vi "Lab Panel V4.82.vi"() -> ()   [LabVIEW 2013] (continued)
                        n628 = Create Folder(path (use dialog)=w999) -> (error out=w998:errorcluster)  [unwired: 2 in, 2 out]
                        n629 = global write "Global 1.vi" "LAB03-1 FILE"(w985) -> ()
                        n630 = call <vilib>:"Clear Errors.vi"("error in (no error)"=w998) -> ()  [unwired: 6 in, 1 out]
                      }
                      frame #1 {
                        n631 = String To Path(string=w1010) -> (path=w1005:path)
                        n632 = TDMS Open(5:FALSE, 6:FALSE, 10:T19."create or replace" ("operation (0:open)"), 11:w1005) -> (0:w1004:errorcluster, 3:→"TDMS LAB03-1":refnum<k34>)  [unwired: 3 in]
                      }
                      frame #2 {
                        n633 = local read "SET LAB03-1"() -> (w1016:T5)
                        n634 = local read "TDMS LAB03-1"() -> (w1027:refnum<k34>)
                        n635 = Build Array("Testers Name", "Description", "Set Test Cycles", "T-Rise minutes", "T-Rise Deg C") -> (w1017:string[])
                        n636 = Unbundle(w1016) -> ("NAME"=w1015:string, "DESCRIPTION"=w1014:string, "CYCLES"=w1013:dbl, "T-RISE mins"=w1012:dbl, "T-RISE deg C"=w1011:dbl)
                        n637 = Number To Decimal String(number=w1013) -> (decimal integer string=w1026:string)  [unwired: 1 in]
                        n638 = Number To Decimal String(number=w1012) -> (decimal integer string=w1025:string)  [unwired: 1 in]
                        n639 = Number To Decimal String(number=w1011) -> (decimal integer string=w1024:string)  [unwired: 1 in]
                        n640 = Build Array(w1015, w1014, w1026, w1025, w1024) -> (w1023:string[])
                        n641 = TDMS Set Properties(5:w1023, 7:w1017, 11:w1027) -> ()  [unwired: 3 in, 4 out]
                      }
                      frame #3 {
                        w1029 = 0.0
                        n642 = local read "DISP LAB03-1"() -> (w1031:T4)
                        n643 = Bundle(cluster=w1031, "CYCLE"=w1029, "MINS"=w1029, "STATUS"="RUN") -> (w1030:T4)
                        n644 = local write "DISP LAB03-1"(w1030) -> ()
                      }
                      frame #4 {
                        n645 = local read "SIG LAB03-1"() -> (w1034:T2)
                        n646 = local read "TEMP START LAB03-1"() -> (w1036:cluster{"TL":dbl, "TN":dbl})
                        n647 = Unbundle(w1034) -> ("Tmp Live"=w1033:dbl, "Tmp Neut"=w1032:dbl)  [unwired: 3 out]
                        n648 = Bundle(cluster=w1036, "TL"=w1033, "TN"=w1032) -> (w1035:cluster{"TL":dbl, "TN":dbl})
                        n649 = local write "TEMP START LAB03-1"(w1035) -> ()
                      }
                    }
                  }
                }
              }
              event "RUN LAB03-2": Value Change {
                n650 = event-data() -> ("NewVal"=w1037:bool)  [unwired: 1 in, 5 out]
                n651 = local write "run lab03-2"(w1037) -> ()
                n652 = case shown="True" w1037 {
                  tunnel: w1043 -> [_ w1076]
                  tunnel: w1042 -> [_ w1075]
                  tunnel: w1040 -> [w1045 w1074]
                  tunnel: w1041 -> [_ w1073]
                  tunnel: w1039 -> [_ w1072]
                  tunnel: [w1044 w1071] -> w1038
                  frame False {
                    # "stop test"
                    n653 = stacked-sequence {
                      tunnel: w1045 -> [w1054 _]
                      tunnel: [w1046 _] -> w1044
                      frame #0 {
                        n654 = local read "DISP LAB03-2"() -> (w1053:T4)
                        n655 = Unbundle(w1053) -> ("CYCLE"=w1051:dbl, "MINS"=w1052:dbl)  [unwired: 1 out]
                        n656 = case shown="\"CYCLE TEST\"" w1054 {
                          tunnel: w1052 -> [_ _ w1061]
                          tunnel: w1051 -> [w1059 w1060 _]
                          tunnel: [w1059 w1060 w1061] -> w1050
                          frame "CHART TEST", Default {
                          }
                          frame "CYCLE TEST" {
                          }
                          frame "T-RISE TEST" {
                          }
                        }
                        n657 = local read "TDMS LAB03-2"() -> (w1058:refnum<k34>)
                        n658 = Build Array("STOPPED") -> (w1055:string[])
                        n659 = Build Array(w1050) -> (w1049:dbl[])
                        n660 = TDMS Write(0:w1058, 5:"TEST RESULT", 7:w1055, 9:w1049) -> (4:w1047:refnum<k34>, 15:w1048:errorcluster)  [unwired: 2 in, 2 out]
                        n661 = TDMS Close(8:w1048, 11:w1047) -> (0:w1046:errorcluster)  [unwired: 1 out]
                      }
                      frame #1 {
                        n662 = local read "DISP LAB03-2"() -> (w1065:T4)
                        n663 = stacked-sequence {
                          tunnel: "LAB03-2" -> [w1067 w1069]
                          frame #0 {
                            n664 = call "sub vi - defrag tdms v1.vi"("panel id"=w1067) -> ("error out"=w1066:errorcluster)  [unwired: 10 in]
                            n665 = local write "data file error"(w1066) -> ()
                          }
                          frame #1 {
                            n666 = call "Save data file to network drive v1.vi"("panel id"=w1069) -> ("network file save error"=w1068:errorcluster)  [unwired: 9 in, 1 out]
                            n667 = local write "RESULT LAB03-2"(FALSE) -> ()
                            n668 = local write "data file error"(w1068) -> ()
                          }
                        }
                        n669 = Bundle(cluster=w1065, "STATUS"="STOP") -> (w1063:T4)  [unwired: 2 in]
                        n670 = local write "DISP LAB03-2"(w1063) -> ()
                      }
                    }
                  }
                  frame True {
                    # "start new test and create test file"
                    n671 = stacked-sequence {
                      seq-local: [w1077 _ _ _ _] -> [_ w1102 _ _ _]
                      tunnel: w1076 -> [w1082 _ _ _ _]
                      tunnel: w1075 -> [w1079 _ _ _ _]
                      tunnel: w1074 -> [w1092 _ _ _ _]
                      tunnel: w1073 -> [w1085 _ _ _ _]
                      tunnel: w1072 -> [w1080 _ _ _ _]
                      tunnel: [_ w1096 _ _ _] -> w1071
                      frame #0 {
                        w1078 = "\\"
                        n672 = local read "SET LAB03-2"() -> (w1087:T5)
                        n673 = case shown="\"T-RISE TEST\"" w1092 {
                          tunnel: ["L03-2-CHART TEST-" "L03-2-CYCLE TEST-" "L03-2-T-RISE TEST-"] -> w1088
                          frame "CHART TEST", Default {
                          }
                          frame "CYCLE TEST" {
                          }
                          frame "T-RISE TEST" {
                          }
                        }
                        n674 = Unbundle(w1087) -> ("DESCRIPTION"=w1086:string)  [unwired: 4 out]
                        n675 = Concatenate Strings(w1082, "\\", w1080, w1078, w1079, w1078) -> (w1089:string)
                        n676 = String To Path(string=w1089) -> (path=w1091:path)
                        n677 = Concatenate Strings(w1089, w1088, w1086, "-", w1085, ".tdms") -> (w1077:string)
                        n678 = Create Folder(path (use dialog)=w1091) -> (error out=w1090:errorcluster)  [unwired: 2 in, 2 out]
                        n679 = global write "Global 1.vi" "LAB03-2 FILE"(w1077) -> ()
                        n680 = call <vilib>:"Clear Errors.vi"("error in (no error)"=w1090) -> ()  [unwired: 6 in, 1 out]
                      }
                      frame #1 {
                        n681 = String To Path(string=w1102) -> (path=w1097:path)
                        n682 = TDMS Open(5:FALSE, 6:FALSE, 10:T19."create or replace" ("operation (0:open)"), 11:w1097) -> (0:w1096:errorcluster, 3:→"TDMS LAB03-2":refnum<k34>)  [unwired: 3 in]
                      }
                      frame #2 {
                        n683 = local read "SET LAB03-2"() -> (w1108:T5)
                        n684 = local read "TDMS LAB03-2"() -> (w1119:refnum<k34>)
                        n685 = Build Array("Testers Name", "Description", "Set Test Cycles", "T-Rise minutes", "T-Rise Deg C") -> (w1109:string[])
                        n686 = Unbundle(w1108) -> ("NAME"=w1107:string, "DESCRIPTION"=w1106:string, "CYCLES"=w1105:dbl, "T-RISE mins"=w1104:dbl, "T-RISE deg C"=w1103:dbl)
                        n687 = Number To Decimal String(number=w1105) -> (decimal integer string=w1118:string)  [unwired: 1 in]
                        n688 = Number To Decimal String(number=w1104) -> (decimal integer string=w1117:string)  [unwired: 1 in]
                        n689 = Number To Decimal String(number=w1103) -> (decimal integer string=w1116:string)  [unwired: 1 in]
                        n690 = Build Array(w1107, w1106, w1118, w1117, w1116) -> (w1115:string[])
                        n691 = TDMS Set Properties(5:w1115, 7:w1109, 11:w1119) -> ()  [unwired: 3 in, 4 out]
                      }
                      frame #3 {
                        w1121 = 0.0
                        n692 = local read "DISP LAB03-2"() -> (w1123:T4)
                        n693 = Bundle(cluster=w1123, "CYCLE"=w1121, "MINS"=w1121, "STATUS"="RUN") -> (w1122:T4)
                        n694 = local write "DISP LAB03-2"(w1122) -> ()
                      }
                      frame #4 {
                        n695 = local read "SIG LAB03-2"() -> (w1126:T2)
                        n696 = local read "TEMP START LAB03-2"() -> (w1128:cluster{"TL":dbl, "TN":dbl})
                        n697 = Unbundle(w1126) -> ("Tmp Live"=w1125:dbl, "Tmp Neut"=w1124:dbl)  [unwired: 3 out]
                        n698 = Bundle(cluster=w1128, "TL"=w1125, "TN"=w1124) -> (w1127:cluster{"TL":dbl, "TN":dbl})
                        n699 = local write "TEMP START LAB03-2"(w1127) -> ()
                      }
                    }
                  }
                }
              }
              event "RUN LAB04-1": Value Change {
                n700 = event-data() -> ("NewVal"=w1129:bool)  [unwired: 1 in, 5 out]
                n701 = local write "run lab04-1"(w1129) -> ()
                n702 = case shown="True" w1129 {
                  tunnel: w1135 -> [_ w1168]
                  tunnel: w1134 -> [_ w1167]
                  tunnel: w1132 -> [w1137 w1166]
                  tunnel: w1133 -> [_ w1165]
                  tunnel: w1131 -> [_ w1164]
                  tunnel: [w1136 w1163] -> w1130
                  frame False {
                    # "stop test"
                    n703 = stacked-sequence {
                      tunnel: w1137 -> [w1146 _]
                      tunnel: [w1138 _] -> w1136
                      frame #0 {
                        n704 = local read "DISP LAB04-1"() -> (w1145:T4)
                        n705 = Unbundle(w1145) -> ("CYCLE"=w1143:dbl, "MINS"=w1144:dbl)  [unwired: 1 out]
                        n706 = case shown="\"CYCLE TEST\"" w1146 {
                          tunnel: w1144 -> [_ _ w1153]
                          tunnel: w1143 -> [w1151 w1152 _]
                          tunnel: [w1151 w1152 w1153] -> w1142
                          frame "CHART TEST", Default {
                          }
                          frame "CYCLE TEST" {
                          }
                          frame "T-RISE TEST" {
                          }
                        }
                        n707 = local read "TDMS LAB04-1"() -> (w1150:refnum<k34>)
                        n708 = Build Array("STOPPED") -> (w1147:string[])
                        n709 = Build Array(w1142) -> (w1141:dbl[])
                        n710 = TDMS Write(0:w1150, 5:"TEST RESULT", 7:w1147, 9:w1141) -> (4:w1139:refnum<k34>, 15:w1140:errorcluster)  [unwired: 2 in, 2 out]
                        n711 = TDMS Close(8:w1140, 11:w1139) -> (0:w1138:errorcluster)  [unwired: 1 out]
                      }
                      frame #1 {
                        n712 = local read "DISP LAB04-1"() -> (w1157:T4)
                        n713 = stacked-sequence {
                          tunnel: "LAB04-1" -> [w1159 w1161]
                          frame #0 {
                            n714 = call "sub vi - defrag tdms v1.vi"("panel id"=w1159) -> ("error out"=w1158:errorcluster)  [unwired: 10 in]
                            n715 = local write "data file error"(w1158) -> ()
                          }
                          frame #1 {
                            n716 = call "Save data file to network drive v1.vi"("panel id"=w1161) -> ("network file save error"=w1160:errorcluster)  [unwired: 9 in, 1 out]
                            n717 = local write "RESULT LAB04-1"(FALSE) -> ()
                            n718 = local write "data file error"(w1160) -> ()
                          }
                        }
                        n719 = Bundle(cluster=w1157, "STATUS"="STOP") -> (w1155:T4)  [unwired: 2 in]
                        n720 = local write "DISP LAB04-1"(w1155) -> ()
                      }
                    }
                  }
                  frame True {
                    # "start new test and create test file"
                    n721 = stacked-sequence {
                      seq-local: [w1169 _ _ _ _] -> [_ w1194 _ _ _]
                      tunnel: w1168 -> [w1174 _ _ _ _]
                      tunnel: w1167 -> [w1170 _ _ _ _]
                      tunnel: w1166 -> [w1184 _ _ _ _]
                      tunnel: w1165 -> [w1177 _ _ _ _]
                      tunnel: w1164 -> [w1172 _ _ _ _]
                      tunnel: [_ w1188 _ _ _] -> w1163
                      frame #0 {
                        w1171 = "\\"
                        n722 = local read "SET LAB04-1"() -> (w1179:T5)
                        n723 = case shown="\"CYCLE TEST\"" w1184 {
                          tunnel: ["L04-1-CHART TEST-" "L04-1-CYCLE TEST-" "L04-1-T-RISE TEST-"] -> w1180
                          frame "CHART TEST", Default {
                          }
                          frame "CYCLE TEST" {
                          }
                          frame "T-RISE TEST" {
                          }
                        }
                        n724 = Unbundle(w1179) -> ("DESCRIPTION"=w1178:string)  [unwired: 4 out]
                        n725 = Concatenate Strings(w1174, "\\", w1172, w1171, w1170, w1171) -> (w1181:string)
                        n726 = String To Path(string=w1181) -> (path=w1183:path)
                        n727 = Concatenate Strings(w1181, w1180, w1178, "-", w1177, ".tdms") -> (w1169:string)
                        n728 = Create Folder(path (use dialog)=w1183) -> (error out=w1182:errorcluster)  [unwired: 2 in, 2 out]
                        n729 = global write "Global 1.vi" "LAB04-1 FILE"(w1169) -> ()
                        n730 = call <vilib>:"Clear Errors.vi"("error in (no error)"=w1182) -> ()  [unwired: 6 in, 1 out]
                      }
                      frame #1 {
                        n731 = String To Path(string=w1194) -> (path=w1189:path)
                        n732 = TDMS Open(5:FALSE, 6:FALSE, 10:T19."create or replace" ("operation (0:open)"), 11:w1189) -> (0:w1188:errorcluster, 3:→"TDMS LAB04-1":refnum<k34>)  [unwired: 3 in]
                      }
                      frame #2 {
                        n733 = local read "SET LAB04-1"() -> (w1200:T5)
                        n734 = local read "TDMS LAB04-1"() -> (w1211:refnum<k34>)
                        n735 = Build Array("Testers Name", "Description", "Set Test Cycles", "T-Rise minutes", "T-Rise Deg C") -> (w1201:string[])
                        n736 = Unbundle(w1200) -> ("NAME"=w1199:string, "DESCRIPTION"=w1198:string, "CYCLES"=w1197:dbl, "T-RISE mins"=w1196:dbl, "T-RISE deg C"=w1195:dbl)
                        n737 = Number To Decimal String(number=w1197) -> (decimal integer string=w1210:string)  [unwired: 1 in]
                        n738 = Number To Decimal String(number=w1196) -> (decimal integer string=w1209:string)  [unwired: 1 in]
                        n739 = Number To Decimal String(number=w1195) -> (decimal integer string=w1208:string)  [unwired: 1 in]
                        n740 = Build Array(w1199, w1198, w1210, w1209, w1208) -> (w1207:string[])
                        n741 = TDMS Set Properties(5:w1207, 7:w1201, 11:w1211) -> ()  [unwired: 3 in, 4 out]
                      }
                      frame #3 {
                        w1213 = 0.0
                        n742 = local read "DISP LAB04-1"() -> (w1215:T4)
                        n743 = Bundle(cluster=w1215, "CYCLE"=w1213, "MINS"=w1213, "STATUS"="RUN") -> (w1214:T4)
                        n744 = local write "DISP LAB04-1"(w1214) -> ()
                      }
                      frame #4 {
                        n745 = local read "SIG LAB04-1"() -> (w1218:T2)
                        n746 = local read "TEMP START LAB04-1"() -> (w1220:cluster{"TL":dbl, "TN":dbl})
                        n747 = Unbundle(w1218) -> ("Tmp Live"=w1217:dbl, "Tmp Neut"=w1216:dbl)  [unwired: 3 out]
                        n748 = Bundle(cluster=w1220, "TL"=w1217, "TN"=w1216) -> (w1219:cluster{"TL":dbl, "TN":dbl})
                        n749 = local write "TEMP START LAB04-1"(w1219) -> ()
                      }
                    }
                  }
                }
              }
              event "RUN LAB04-2": Value Change {
                n750 = event-data() -> ("NewVal"=w1221:bool)  [unwired: 1 in, 5 out]
                n751 = local write "run lab04-2"(w1221) -> ()
                n752 = case shown="True" w1221 {
                  tunnel: w1227 -> [_ w1260]
                  tunnel: w1226 -> [_ w1259]
                  tunnel: w1224 -> [w1229 w1258]
                  tunnel: w1225 -> [_ w1257]
                  tunnel: w1223 -> [_ w1256]
                  tunnel: [w1228 w1255] -> w1222
                  frame False {
                    # "stop test"
                    n753 = stacked-sequence {
                      tunnel: w1229 -> [w1238 _]
                      tunnel: [w1230 _] -> w1228
                      frame #0 {
                        n754 = local read "DISP LAB04-2"() -> (w1237:T4)
                        n755 = Unbundle(w1237) -> ("CYCLE"=w1235:dbl, "MINS"=w1236:dbl)  [unwired: 1 out]
                        n756 = case shown="\"CYCLE TEST\"" w1238 {
                          tunnel: w1236 -> [_ _ w1245]
                          tunnel: w1235 -> [w1243 w1244 _]
                          tunnel: [w1243 w1244 w1245] -> w1234
                          frame "CHART TEST", Default {
                          }
                          frame "CYCLE TEST" {
                          }
                          frame "T-RISE TEST" {
                          }
                        }
                        n757 = local read "TDMS LAB04-2"() -> (w1242:refnum<k34>)
                        n758 = Build Array("STOPPED") -> (w1239:string[])
                        n759 = Build Array(w1234) -> (w1233:dbl[])
                        n760 = TDMS Write(0:w1242, 5:"TEST RESULT", 7:w1239, 9:w1233) -> (4:w1231:refnum<k34>, 15:w1232:errorcluster)  [unwired: 2 in, 2 out]
                        n761 = TDMS Close(8:w1232, 11:w1231) -> (0:w1230:errorcluster)  [unwired: 1 out]
                      }
                      frame #1 {
                        n762 = local read "DISP LAB04-2"() -> (w1249:T4)
                        n763 = stacked-sequence {
                          tunnel: "LAB04-2" -> [w1251 w1253]
                          frame #0 {
                            n764 = call "sub vi - defrag tdms v1.vi"("panel id"=w1251) -> ("error out"=w1250:errorcluster)  [unwired: 10 in]
                            n765 = local write "data file error"(w1250) -> ()
                          }
                          frame #1 {
                            n766 = call "Save data file to network drive v1.vi"("panel id"=w1253) -> ("network file save error"=w1252:errorcluster)  [unwired: 9 in, 1 out]
                            n767 = local write "RESULT LAB04-2"(FALSE) -> ()
                            n768 = local write "data file error"(w1252) -> ()
                          }
                        }
                        n769 = Bundle(cluster=w1249, "STATUS"="STOP") -> (w1247:T4)  [unwired: 2 in]
                        n770 = local write "DISP LAB04-2"(w1247) -> ()
                      }
                    }
                  }
                  frame True {
                    # "start new test and create test file"
                    n771 = stacked-sequence {
                      seq-local: [w1261 _ _ _ _] -> [_ w1286 _ _ _]
                      tunnel: w1260 -> [w1266 _ _ _ _]
                      tunnel: w1259 -> [w1262 _ _ _ _]
                      tunnel: w1258 -> [w1276 _ _ _ _]
                      tunnel: w1257 -> [w1269 _ _ _ _]
                      tunnel: w1256 -> [w1264 _ _ _ _]
                      tunnel: [_ w1280 _ _ _] -> w1255
                      frame #0 {
                        w1263 = "\\"
                        n772 = local read "SET LAB04-2"() -> (w1271:T5)
                        n773 = case shown="\"CHART TEST\", Default" w1276 {
                          tunnel: ["L04-2-CHART TEST-" "L04-2-CYCLE TEST-" "L04-2-T-RISE TEST-"] -> w1272
                          frame "CHART TEST", Default {
                          }
                          frame "CYCLE TEST" {
                          }
                          frame "T-RISE TEST" {
                          }
                        }
                        n774 = Unbundle(w1271) -> ("DESCRIPTION"=w1270:string)  [unwired: 4 out]
                        n775 = Concatenate Strings(w1266, "\\", w1264, w1263, w1262, w1263) -> (w1273:string)
                        n776 = String To Path(string=w1273) -> (path=w1275:path)
                        n777 = Concatenate Strings(w1273, w1272, w1270, "-", w1269, ".tdms") -> (w1261:string)
                        n778 = Create Folder(path (use dialog)=w1275) -> (error out=w1274:errorcluster)  [unwired: 2 in, 2 out]
                        n779 = global write "Global 1.vi" "LAB04-2 FILE"(w1261) -> ()
                        n780 = call <vilib>:"Clear Errors.vi"("error in (no error)"=w1274) -> ()  [unwired: 6 in, 1 out]
                      }
                      frame #1 {
                        n781 = String To Path(string=w1286) -> (path=w1281:path)
                        n782 = TDMS Open(5:FALSE, 6:FALSE, 10:T19."create or replace" ("operation (0:open)"), 11:w1281) -> (0:w1280:errorcluster, 3:→"TDMS LAB04-2":refnum<k34>)  [unwired: 3 in]
                      }
                      frame #2 {
                        n783 = local read "SET LAB04-2"() -> (w1292:T5)
                        n784 = local read "TDMS LAB04-2"() -> (w1303:refnum<k34>)
                        n785 = Build Array("Testers Name", "Description", "Set Test Cycles", "T-Rise minutes", "T-Rise Deg C") -> (w1293:string[])
                        n786 = Unbundle(w1292) -> ("NAME"=w1291:string, "DESCRIPTION"=w1290:string, "CYCLES"=w1289:dbl, "T-RISE mins"=w1288:dbl, "T-RISE deg C"=w1287:dbl)
                        n787 = Number To Decimal String(number=w1289) -> (decimal integer string=w1302:string)  [unwired: 1 in]
                        n788 = Number To Decimal String(number=w1288) -> (decimal integer string=w1301:string)  [unwired: 1 in]
                        n789 = Number To Decimal String(number=w1287) -> (decimal integer string=w1300:string)  [unwired: 1 in]
                        n790 = Build Array(w1291, w1290, w1302, w1301, w1300) -> (w1299:string[])
                        n791 = TDMS Set Properties(5:w1299, 7:w1293, 11:w1303) -> ()  [unwired: 3 in, 4 out]
                      }
                      frame #3 {
                        w1305 = 0.0
                        n792 = local read "DISP LAB04-2"() -> (w1307:T4)
                        n793 = Bundle(cluster=w1307, "CYCLE"=w1305, "MINS"=w1305, "STATUS"="RUN") -> (w1306:T4)
                        n794 = local write "DISP LAB04-2"(w1306) -> ()
                      }
                      frame #4 {
                        n795 = local read "SIG LAB04-2"() -> (w1310:T2)
                        n796 = local read "TEMP START LAB04-2"() -> (w1312:cluster{"TL":dbl, "TN":dbl})
                        n797 = Unbundle(w1310) -> ("Tmp Live"=w1309:dbl, "Tmp Neut"=w1308:dbl)  [unwired: 3 out]
                        n798 = Bundle(cluster=w1312, "TL"=w1309, "TN"=w1308) -> (w1311:cluster{"TL":dbl, "TN":dbl})
                        n799 = local write "TEMP START LAB04-2"(w1311) -> ()
                      }
                    }
                  }
                }
              }
              event "RUN LAB05-1": Value Change {
                n800 = event-data() -> ("NewVal"=w1313:bool)  [unwired: 1 in, 5 out]
                n801 = local write "run lab05-1"(w1313) -> ()
                n802 = case shown="True" w1313 {
                  tunnel: w1319 -> [_ w1352]
                  tunnel: w1318 -> [_ w1351]
                  tunnel: w1316 -> [w1321 w1350]
                  tunnel: w1317 -> [_ w1349]
                  tunnel: w1315 -> [_ w1348]
                  tunnel: [w1320 w1347] -> w1314
                  frame False {
                    # "stop test"
                    n803 = stacked-sequence {
                      tunnel: w1321 -> [w1330 _]
                      tunnel: [w1322 _] -> w1320
                      frame #0 {
                        n804 = local read "DISP LAB05-1"() -> (w1329:T4)
                        n805 = Unbundle(w1329) -> ("CYCLE"=w1327:dbl, "MINS"=w1328:dbl)  [unwired: 1 out]
                        n806 = case shown="\"CYCLE TEST\"" w1330 {
                          tunnel: w1328 -> [_ _ w1337]
                          tunnel: w1327 -> [w1335 w1336 _]
                          tunnel: [w1335 w1336 w1337] -> w1326
                          frame "CHART TEST", Default {
                          }
                          frame "CYCLE TEST" {
                          }
                          frame "T-RISE TEST" {
                          }
                        }
                        n807 = local read "TDMS LAB05-1"() -> (w1334:refnum<k34>)
                        n808 = Build Array("STOPPED") -> (w1331:string[])
                        n809 = Build Array(w1326) -> (w1325:dbl[])
                        n810 = TDMS Write(0:w1334, 5:"TEST RESULT", 7:w1331, 9:w1325) -> (4:w1323:refnum<k34>, 15:w1324:errorcluster)  [unwired: 2 in, 2 out]
                        n811 = TDMS Close(8:w1324, 11:w1323) -> (0:w1322:errorcluster)  [unwired: 1 out]
                      }
                      frame #1 {
                        n812 = local read "DISP LAB05-1"() -> (w1341:T4)
                        n813 = stacked-sequence {
                          tunnel: "LAB05-1" -> [w1343 w1345]
                          frame #0 {
                            n814 = call "sub vi - defrag tdms v1.vi"("panel id"=w1343) -> ("error out"=w1342:errorcluster)  [unwired: 10 in]
                            n815 = local write "data file error"(w1342) -> ()
                          }
                          frame #1 {
                            n816 = call "Save data file to network drive v1.vi"("panel id"=w1345) -> ("network file save error"=w1344:errorcluster)  [unwired: 9 in, 1 out]
                            n817 = local write "RESULT LAB05-1"(FALSE) -> ()
                            n818 = local write "data file error"(w1344) -> ()
                          }
                        }
                        n819 = Bundle(cluster=w1341, "STATUS"="STOP") -> (w1339:T4)  [unwired: 2 in]
                        n820 = local write "DISP LAB05-1"(w1339) -> ()
                      }
                    }
                  }
                  frame True {
                    # "start new test and create test file"
                    n821 = stacked-sequence {
                      seq-local: [w1353 _ _ _ _] -> [_ w1378 _ _ _]
                      tunnel: w1352 -> [w1358 _ _ _ _]
                      tunnel: w1351 -> [w1354 _ _ _ _]
                      tunnel: w1350 -> [w1368 _ _ _ _]
                      tunnel: w1349 -> [w1361 _ _ _ _]
                      tunnel: w1348 -> [w1356 _ _ _ _]
                      tunnel: [_ w1372 _ _ _] -> w1347
                      frame #0 {
                        w1355 = "\\"
                        n822 = local read "SET LAB05-1"() -> (w1363:T5)
                        n823 = case shown="\"CYCLE TEST\"" w1368 {
                          tunnel: ["L05-1-CHART TEST-" "L05-1-CYCLE TEST-" "L05-1-T-RISE TEST-"] -> w1364
                          frame "CHART TEST", Default {
                          }
                          frame "CYCLE TEST" {
                          }
                          frame "T-RISE TEST" {
                          }
                        }
                        n824 = Unbundle(w1363) -> ("DESCRIPTION"=w1362:string)  [unwired: 4 out]
                        n825 = Concatenate Strings(w1358, "\\", w1356, w1355, w1354, w1355) -> (w1365:string)
                        n826 = String To Path(string=w1365) -> (path=w1367:path)
                        n827 = Concatenate Strings(w1365, w1364, w1362, "-", w1361, ".tdms") -> (w1353:string)
                        n828 = Create Folder(path (use dialog)=w1367) -> (error out=w1366:errorcluster)  [unwired: 2 in, 2 out]
                        n829 = global write "Global 1.vi" "LAB05-1 FILE"(w1353) -> ()
                        n830 = call <vilib>:"Clear Errors.vi"("error in (no error)"=w1366) -> ()  [unwired: 6 in, 1 out]
                      }
                      frame #1 {
                        n831 = String To Path(string=w1378) -> (path=w1373:path)
                        n832 = TDMS Open(5:FALSE, 6:FALSE, 10:T19."create or replace" ("operation (0:open)"), 11:w1373) -> (0:w1372:errorcluster, 3:→"TDMS LAB05-1":refnum<k34>)  [unwired: 3 in]
                      }
                      frame #2 {
                        n833 = local read "SET LAB05-1"() -> (w1384:T5)
                        n834 = local read "TDMS LAB05-1"() -> (w1395:refnum<k34>)
                        n835 = Build Array("Testers Name", "Description", "Set Test Cycles", "T-Rise minutes", "T-Rise Deg C") -> (w1385:string[])
                        n836 = Unbundle(w1384) -> ("NAME"=w1383:string, "DESCRIPTION"=w1382:string, "CYCLES"=w1381:dbl, "T-RISE mins"=w1380:dbl, "T-RISE deg C"=w1379:dbl)
                        n837 = Number To Decimal String(number=w1381) -> (decimal integer string=w1394:string)  [unwired: 1 in]
                        n838 = Number To Decimal String(number=w1380) -> (decimal integer string=w1393:string)  [unwired: 1 in]
                        n839 = Number To Decimal String(number=w1379) -> (decimal integer string=w1392:string)  [unwired: 1 in]
                        n840 = Build Array(w1383, w1382, w1394, w1393, w1392) -> (w1391:string[])
                        n841 = TDMS Set Properties(5:w1391, 7:w1385, 11:w1395) -> ()  [unwired: 3 in, 4 out]
                      }
                      frame #3 {
                        w1397 = 0.0
                        n842 = local read "DISP LAB05-1"() -> (w1399:T4)
                        n843 = Bundle(cluster=w1399, "CYCLE"=w1397, "MINS"=w1397, "STATUS"="RUN") -> (w1398:T4)
                        n844 = local write "DISP LAB05-1"(w1398) -> ()
                      }
                      frame #4 {
                        n845 = local read "SIG LAB05-1"() -> (w1402:T2)
                        n846 = local read "TEMP START LAB05-1"() -> (w1404:cluster{"TL":dbl, "TN":dbl})
                        n847 = Unbundle(w1402) -> ("Tmp Live"=w1401:dbl, "Tmp Neut"=w1400:dbl)  [unwired: 3 out]
                        n848 = Bundle(cluster=w1404, "TL"=w1401, "TN"=w1400) -> (w1403:cluster{"TL":dbl, "TN":dbl})
                        n849 = local write "TEMP START LAB05-1"(w1403) -> ()
                      }
                    }
                  }
                }
              }
              event "RUN LAB05-2": Value Change {
                n850 = event-data() -> ("NewVal"=w1405:bool)  [unwired: 1 in, 5 out]
                n851 = local write "run lab05-2"(w1405) -> ()
                n852 = case shown="True" w1405 {
                  tunnel: w1411 -> [_ w1444]
                  tunnel: w1410 -> [_ w1443]
                  tunnel: w1408 -> [w1413 w1442]
                  tunnel: w1409 -> [_ w1441]
                  tunnel: w1407 -> [_ w1440]
                  tunnel: [w1412 w1439] -> w1406
                  frame False {
                    # "stop test"
                    n853 = stacked-sequence {
                      tunnel: w1413 -> [w1422 _]
                      tunnel: [w1414 _] -> w1412
                      frame #0 {
                        n854 = local read "DISP LAB05-2"() -> (w1421:T4)
                        n855 = Unbundle(w1421) -> ("CYCLE"=w1419:dbl, "MINS"=w1420:dbl)  [unwired: 1 out]
                        n856 = case shown="\"CYCLE TEST\"" w1422 {
                          tunnel: w1420 -> [_ _ w1429]
                          tunnel: w1419 -> [w1427 w1428 _]
                          tunnel: [w1427 w1428 w1429] -> w1418
                          frame "CHART TEST", Default {
                          }
                          frame "CYCLE TEST" {
                          }
                          frame "T-RISE TEST" {
                          }
                        }
                        n857 = local read "TDMS LAB05-2"() -> (w1426:refnum<k34>)
                        n858 = Build Array("STOPPED") -> (w1423:string[])
                        n859 = Build Array(w1418) -> (w1417:dbl[])
                        n860 = TDMS Write(0:w1426, 5:"TEST RESULT", 7:w1423, 9:w1417) -> (4:w1415:refnum<k34>, 15:w1416:errorcluster)  [unwired: 2 in, 2 out]
                        n861 = TDMS Close(8:w1416, 11:w1415) -> (0:w1414:errorcluster)  [unwired: 1 out]
                      }
                      frame #1 {
                        n862 = local read "DISP LAB05-2"() -> (w1433:T4)
                        n863 = stacked-sequence {
                          tunnel: "LAB05-2" -> [w1435 w1437]
                          frame #0 {
                            n864 = call "sub vi - defrag tdms v1.vi"("panel id"=w1435) -> ("error out"=w1434:errorcluster)  [unwired: 10 in]
                            n865 = local write "data file error"(w1434) -> ()
                          }
                          frame #1 {
                            n866 = local write "RESULT LAB05-2"(FALSE) -> ()
                            n867 = call "Save data file to network drive v1.vi"("panel id"=w1437) -> ("network file save error"=w1436:errorcluster)  [unwired: 9 in, 1 out]
                            n868 = local write "data file error"(w1436) -> ()
                          }
                        }
                        n869 = Bundle(cluster=w1433, "STATUS"="STOP") -> (w1431:T4)  [unwired: 2 in]
                        n870 = local write "DISP LAB05-2"(w1431) -> ()
                      }
                    }
                  }
                  frame True {
                    # "start new test and create test file"
                    n871 = stacked-sequence {
                      seq-local: [w1445 _ _ _ _] -> [_ w1470 _ _ _]
                      tunnel: w1444 -> [w1450 _ _ _ _]
                      tunnel: w1443 -> [w1446 _ _ _ _]
                      tunnel: w1442 -> [w1460 _ _ _ _]
                      tunnel: w1441 -> [w1453 _ _ _ _]
                      tunnel: w1440 -> [w1448 _ _ _ _]
                      tunnel: [_ w1464 _ _ _] -> w1439
                      frame #0 {
                        w1447 = "\\"
                        n872 = local read "SET LAB05-2"() -> (w1455:T5)
                        n873 = case shown="\"CYCLE TEST\"" w1460 {
                          tunnel: ["L05-2-CHART TEST-" "L05-2-CYCLE TEST-" "L05-2-T-RISE TEST-"] -> w1456
                          frame "CHART TEST", Default {
                          }
                          frame "CYCLE TEST" {
                          }
                          frame "T-RISE TEST" {
                          }
                        }
                        n874 = Unbundle(w1455) -> ("DESCRIPTION"=w1454:string)  [unwired: 4 out]
                        n875 = Concatenate Strings(w1450, "\\", w1448, w1447, w1446, w1447) -> (w1457:string)
                        n876 = String To Path(string=w1457) -> (path=w1459:path)
                        n877 = Concatenate Strings(w1457, w1456, w1454, "-", w1453, ".tdms") -> (w1445:string)
                        n878 = Create Folder(path (use dialog)=w1459) -> (error out=w1458:errorcluster)  [unwired: 2 in, 2 out]
                        n879 = global write "Global 1.vi" "LAB05-2 FILE"(w1445) -> ()
                        n880 = call <vilib>:"Clear Errors.vi"("error in (no error)"=w1458) -> ()  [unwired: 6 in, 1 out]
                      }
                      frame #1 {
                        n881 = String To Path(string=w1470) -> (path=w1465:path)
                        n882 = TDMS Open(5:FALSE, 6:FALSE, 10:T19."create or replace" ("operation (0:open)"), 11:w1465) -> (0:w1464:errorcluster, 3:→"TDMS LAB05-2":refnum<k34>)  [unwired: 3 in]
                      }
                      frame #2 {
                        n883 = local read "SET LAB05-2"() -> (w1476:T5)
                        n884 = local read "TDMS LAB05-2"() -> (w1487:refnum<k34>)
                        n885 = Build Array("Testers Name", "Description", "Set Test Cycles", "T-Rise minutes", "T-Rise Deg C") -> (w1477:string[])
                        n886 = Unbundle(w1476) -> ("NAME"=w1475:string, "DESCRIPTION"=w1474:string, "CYCLES"=w1473:dbl, "T-RISE mins"=w1472:dbl, "T-RISE deg C"=w1471:dbl)
                        n887 = Number To Decimal String(number=w1473) -> (decimal integer string=w1486:string)  [unwired: 1 in]
                        n888 = Number To Decimal String(number=w1472) -> (decimal integer string=w1485:string)  [unwired: 1 in]
                        n889 = Number To Decimal String(number=w1471) -> (decimal integer string=w1484:string)  [unwired: 1 in]
                        n890 = Build Array(w1475, w1474, w1486, w1485, w1484) -> (w1483:string[])
                        n891 = TDMS Set Properties(5:w1483, 7:w1477, 11:w1487) -> ()  [unwired: 3 in, 4 out]
                      }
                      frame #3 {
                        w1489 = 0.0
                        n892 = local read "DISP LAB05-2"() -> (w1491:T4)
                        n893 = Bundle(cluster=w1491, "CYCLE"=w1489, "MINS"=w1489, "STATUS"="RUN") -> (w1490:T4)
                        n894 = local write "DISP LAB05-2"(w1490) -> ()
                      }
                      frame #4 {
                        n895 = local read "SIG LAB05-2"() -> (w1494:T2)
                        n896 = local read "TEMP START LAB05-2"() -> (w1496:cluster{"TL":dbl, "TN":dbl})
                        n897 = Unbundle(w1494) -> ("Tmp Live"=w1493:dbl, "Tmp Neut"=w1492:dbl)  [unwired: 3 out]
                        n898 = Bundle(cluster=w1496, "TL"=w1493, "TN"=w1492) -> (w1495:cluster{"TL":dbl, "TN":dbl})
                        n899 = local write "TEMP START LAB05-2"(w1495) -> ()
                      }
                    }
                  }
                }
              }
            }
            n900 = local write "data file error"(w548) -> ()
          }
          frame #4 {
            # "check if test cycles reached for cycle tests, if so then test pass"
            n901 = stacked-sequence {
              tunnel: w1516 -> [_ _ _ _ _ _ _ _ _ _]
              tunnel: w1515 -> [_ _ _ _ _ _ _ _ _ _]
              tunnel: w1514 -> [_ _ _ _ _ _ _ _ _ _]
              tunnel: w1513 -> [_ _ _ _ _ _ _ _ _ _]
              tunnel: w1512 -> [_ _ _ _ _ _ _ _ _ _]
              tunnel: w1511 -> [_ _ _ _ _ _ _ _ _ _]
              tunnel: w1510 -> [_ _ _ _ _ _ _ _ _ _]
              tunnel: w1509 -> [_ _ _ _ _ _ _ _ _ _]
              tunnel: w1508 -> [_ _ _ _ _ _ _ _ _ _]
              tunnel: w1507 -> [_ _ _ _ _ _ _ _ _ _]
              tunnel: w1506 -> [w1522 _ _ _ _ _ _ _ _ _]
              tunnel: w1505 -> [_ w1557 _ _ _ _ _ _ _ _]
              tunnel: w1504 -> [_ _ w1597 _ _ _ _ _ _ _]
              tunnel: w1503 -> [_ _ _ w1637 _ _ _ _ _ _]
              tunnel: w1502 -> [_ _ _ _ w1677 _ _ _ _ _]
              tunnel: w1501 -> [_ _ _ _ _ w1717 _ _ _ _]
              tunnel: w1500 -> [_ _ _ _ _ _ w1757 _ _ _]
              tunnel: w1499 -> [_ _ _ _ _ _ _ w1797 _ _]
              tunnel: w1498 -> [_ _ _ _ _ _ _ _ w1837 _]
              tunnel: w1497 -> [_ _ _ _ _ _ _ _ _ w1877]
              frame #0 {
                # "LAB01-1"
                n902 = Less?(x=w1522, y=2) -> (x < y?=w1520:bool)
                n903 = local read "DISP LAB01-1"() -> (w1523:T4)
                n904 = Unbundle(w1523) -> ("STATUS"=w1517:string)  [unwired: 2 out]
                n905 = Equal?(x=w1517, y="RUN") -> (x = y?=w1519:bool)
                n906 = And(x=w1519, y=w1520) -> (x .and. y?=w1518:bool)
                n907 = case shown="True" w1518 {
                  tunnel: w1523 -> [_ w1528]
                  tunnel: w1522 -> [_ w1532]
                  frame False {
                  }
                  frame True {
                    n908 = local read "SET LAB01-1"() -> (w1534:T5)
                    n909 = local read "TDMS LAB01-1"() -> (w1527:refnum<k34>)
                    n910 = Unbundle(w1534) -> ("CYCLES"=w1525:dbl, "T-RISE mins"=w1531:dbl)  [unwired: 3 out]
                    n911 = case shown="\"CYCLE TEST\"" w1532 {
                      tunnel: w1531 -> [_ _ w1541]
                      tunnel: [w1536 w1538 w1541] -> w1530
                      tunnel: w1525 -> [w1536 w1538 _]
                      tunnel: ["CHART PASS" "CYCLE PASS" "T-RISE PASS"] -> w1529
                      frame "CHART TEST", Default {
                      }
                      frame "CYCLE TEST" {
                      }
                      frame "T-RISE TEST" {
                      }
                    }
                    n912 = Unbundle(w1528) -> ("CYCLE"=w1533:dbl)  [unwired: 2 out]
                    n913 = Increment(x=w1525) -> (x+1=w1526:dbl)
                    n914 = Greater Or Equal?(x=w1533, y=w1526) -> (x >= y?=w1535:bool)
                    n915 = case shown="True" w1535 {
                      tunnel: w1530 -> [w1545 _]
                      tunnel: w1529 -> [w1544 _]
                      tunnel: w1528 -> [w1543 _]
                      tunnel: w1527 -> [w1542 _]
                      frame True {
                        n916 = stacked-sequence {
                          tunnel: w1545 -> [w1549 _]
                          tunnel: w1544 -> [w1547 w1553]
                          tunnel: w1543 -> [_ w1556]
                          tunnel: w1542 -> [w1546 _]
                          frame #0 {
                            n917 = Build Array(w1547) -> (w1550:string[])
                            n918 = Build Array(w1549) -> (w1548:dbl[])
                            n919 = TDMS Write(0:w1546, 5:"TEST PASS", 7:w1550, 9:w1548) -> (15:w1552:errorcluster)  [unwired: 2 in, 3 out]
                            n920 = local write "data file error"(w1552) -> ()
                          }
                          frame #1 {
                            n921 = Bundle(cluster=w1556, "STATUS"=w1553) -> (w1554:T4)  [unwired: 2 in]
                            n922 = local write "RESULT LAB01-1"(TRUE) -> ()
                            n923 = local write "DISP LAB01-1"(w1554) -> ()
                          }
                        }
                      }
                      frame False {
                      }
                    }
                  }
                }
              }
              frame #1 {
                # "LAB01-2"
                n924 = Less?(x=w1557, y=2) -> (x < y?=w1560:bool)
                n925 = local read "DISP LAB01-2"() -> (w1562:T4)
                n926 = Unbundle(w1562) -> ("STATUS"=w1563:string)  [unwired: 2 out]
                n927 = Equal?(x=w1563, y="RUN") -> (x = y?=w1559:bool)
                n928 = And(x=w1559, y=w1560) -> (x .and. y?=w1558:bool)
                n929 = case shown="True" w1558 {
                  tunnel: w1562 -> [_ w1568]
                  tunnel: w1557 -> [_ w1572]
                  frame False {
                  }
                  frame True {
                    n930 = local read "SET LAB01-2"() -> (w1574:T5)
                    n931 = local read "TDMS LAB01-2"() -> (w1567:refnum<k34>)
                    n932 = Unbundle(w1574) -> ("CYCLES"=w1565:dbl, "T-RISE mins"=w1571:dbl)  [unwired: 3 out]
                    n933 = case shown="\"T-RISE TEST\"" w1572 {
                      tunnel: w1571 -> [_ _ w1581]
                      tunnel: [w1576 w1578 w1581] -> w1570
                      tunnel: w1565 -> [w1576 w1578 _]
                      tunnel: ["CHART PASS" "CYCLE PASS" "T-RISE PASS"] -> w1569
                      frame "CHART TEST", Default {
                      }
                      frame "CYCLE TEST" {
                      }
                      frame "T-RISE TEST" {
                      }
                    }
                    n934 = Unbundle(w1568) -> ("CYCLE"=w1573:dbl)  [unwired: 2 out]
                    n935 = Increment(x=w1565) -> (x+1=w1566:dbl)
                    n936 = Greater Or Equal?(x=w1573, y=w1566) -> (x >= y?=w1575:bool)
                    n937 = case shown="True" w1575 {
                      tunnel: w1570 -> [w1585 _]
                      tunnel: w1569 -> [w1584 _]
                      tunnel: w1568 -> [w1583 _]
                      tunnel: w1567 -> [w1582 _]
                      frame True {
                        n938 = stacked-sequence {
                          tunnel: w1585 -> [w1589 _]
                          tunnel: w1584 -> [w1587 w1593]
                          tunnel: w1583 -> [_ w1596]
                          tunnel: w1582 -> [w1586 _]
                          frame #0 {
                            n939 = Build Array(w1587) -> (w1590:string[])
                            n940 = Build Array(w1589) -> (w1588:dbl[])
                            n941 = TDMS Write(0:w1586, 5:"TEST PASS", 7:w1590, 9:w1588) -> (15:w1592:errorcluster)  [unwired: 2 in, 3 out]
                            n942 = local write "data file error"(w1592) -> ()
                          }
                          frame #1 {
                            n943 = Bundle(cluster=w1596, "STATUS"=w1593) -> (w1594:T4)  [unwired: 2 in]
                            n944 = local write "RESULT LAB01-2"(TRUE) -> ()
                            n945 = local write "DISP LAB01-2"(w1594) -> ()
                          }
                        }
                      }
                      frame False {
                      }
                    }
                  }
                }
              }
              frame #2 {
                # "LAB02-1"
                n946 = Less?(x=w1597, y=2) -> (x < y?=w1600:bool)
                n947 = local read "DISP LAB02-1"() -> (w1602:T4)
                n948 = Unbundle(w1602) -> ("STATUS"=w1603:string)  [unwired: 2 out]
                n949 = Equal?(x=w1603, y="RUN") -> (x = y?=w1599:bool)
                n950 = And(x=w1599, y=w1600) -> (x .and. y?=w1598:bool)
                n951 = case shown="True" w1598 {
                  tunnel: w1602 -> [_ w1608]
                  tunnel: w1597 -> [_ w1612]
                  frame False {
                  }
                  frame True {
                    n952 = local read "SET LAB02-1"() -> (w1614:T5)
                    n953 = local read "TDMS LAB02-1"() -> (w1607:refnum<k34>)
                    n954 = Unbundle(w1608) -> ("CYCLE"=w1613:dbl)  [unwired: 2 out]
                    n955 = Unbundle(w1614) -> ("CYCLES"=w1605:dbl, "T-RISE mins"=w1611:dbl)  [unwired: 3 out]
                    n956 = case shown="\"T-RISE TEST\"" w1612 {
                      tunnel: w1611 -> [_ _ w1621]
                      tunnel: [w1616 w1618 w1621] -> w1610
                      tunnel: w1605 -> [w1616 w1618 _]
                      tunnel: ["CHART PASS" "CYCLE PASS" "T-RISE PASS"] -> w1609
                      frame "CHART TEST", Default {
                      }
                      frame "CYCLE TEST" {
                      }
                      frame "T-RISE TEST" {
                      }
                    }
                    n957 = Increment(x=w1605) -> (x+1=w1606:dbl)
                    n958 = Greater Or Equal?(x=w1613, y=w1606) -> (x >= y?=w1615:bool)
                    n959 = case shown="True" w1615 {
                      tunnel: w1610 -> [w1625 _]
                      tunnel: w1609 -> [w1624 _]
                      tunnel: w1608 -> [w1623 _]
                      tunnel: w1607 -> [w1622 _]
                      frame True {
                        n960 = stacked-sequence {
                          tunnel: w1625 -> [w1629 _]
                          tunnel: w1624 -> [w1627 w1633]
                          tunnel: w1623 -> [_ w1636]
                          tunnel: w1622 -> [w1626 _]
                          frame #0 {
                            n961 = Build Array(w1627) -> (w1630:string[])
                            n962 = Build Array(w1629) -> (w1628:dbl[])
                            n963 = TDMS Write(0:w1626, 5:"TEST PASS", 7:w1630, 9:w1628) -> (15:w1632:errorcluster)  [unwired: 2 in, 3 out]
                            n964 = local write "data file error"(w1632) -> ()
                          }
                          frame #1 {
                            n965 = Bundle(cluster=w1636, "STATUS"=w1633) -> (w1634:T4)  [unwired: 2 in]
                            n966 = local write "RESULT LAB02-1"(TRUE) -> ()
                            n967 = local write "DISP LAB02-1"(w1634) -> ()
                          }
                        }
                      }
                      frame False {
                      }
                    }
                  }
                }
              }
              frame #3 {
                # "LAB02-2"
